vi "PH_BL-Master.get class of status subscriber.vi"(0 "GUI Ref":refnum<vi>, 1 "Ref Switch Instances":refnum<vi>, 2 "Ref BB Instances":refnum<vi>, 3 "Ref 6P Switch Instances":refnum<vi>, 4 "Ref Switch GUI Instances":refnum<vi>, 5 "Ref Switch and 6P State Instances":refnum<vi>, 7 "Force Sensor Instances":refnum<vi>) -> (17 "Status Subscriber Class":T1)   [LabVIEW 2014, in "PH_BL-Master.lvlib"]
uses:
  PH_BL-Master.lvlib
  PH_BL-Master.Status Subscriber Class.ctl
  PH_Basics/PH_Common/PH_Common.lvlib
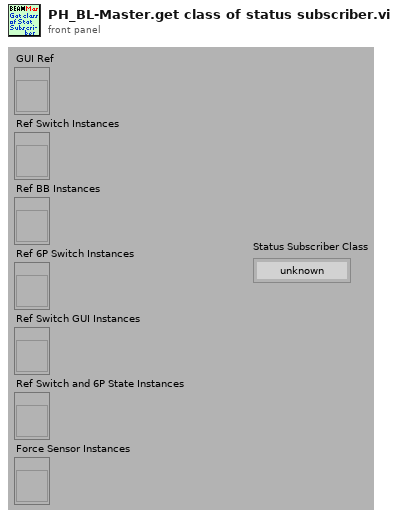
[diagram p1: front panel]
types:
  T1 = typedef "PH_BL-Master.lvlib/PH_BL-Master.Status Subscriber Class.ctl" = enum16{"unknown", "Switch", "BB", "6P Switch", "Switch GUI", "Switch and 6P State", "Force Sensor"}
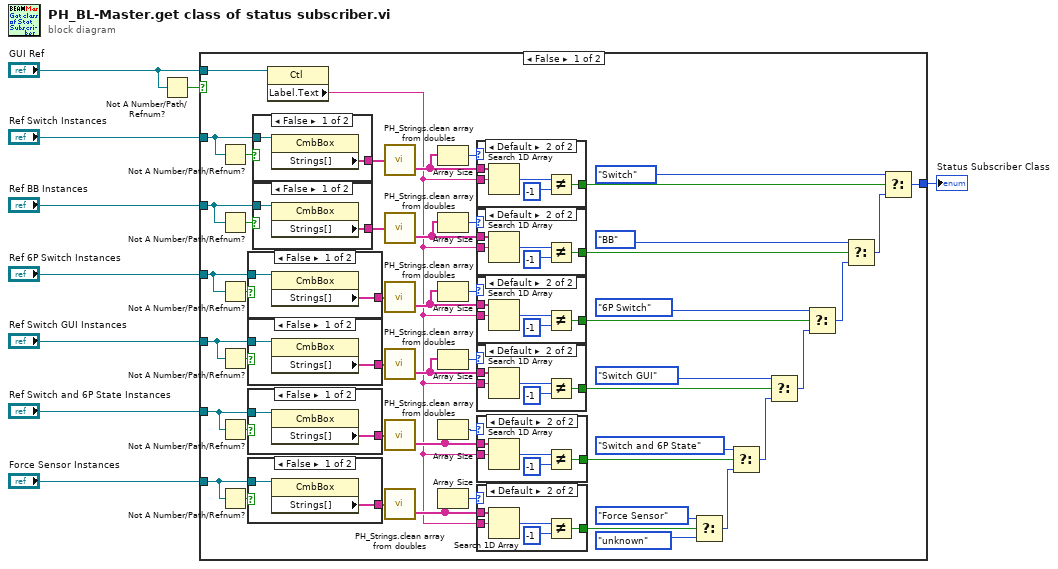
[diagram p0: block diagram]
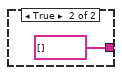
[diagram p2: hidden frame]
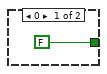
[diagram p3: hidden frame]
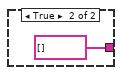
[diagram p4: hidden frame]
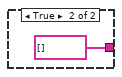
[diagram p5: hidden frame]
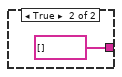
[diagram p6: hidden frame]
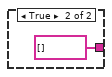
[diagram p7: hidden frame]
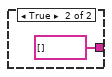
[diagram p8: hidden frame]
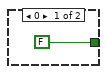
[diagram p9: hidden frame]
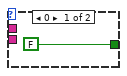
[diagram p10: hidden frame]
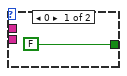
[diagram p11: hidden frame]
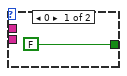
[diagram p12: hidden frame]
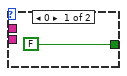
[diagram p13: hidden frame]
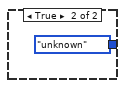
[diagram p14: hidden frame]
diagram:
  n1 = Not A Number/Path/Refnum?(number/path/refnum="GUI Ref") -> (NaN/Path/Refnum?=w2:bool)
  n2 = case shown="False" w2 {
    tunnel: "GUI Ref" -> [w59 _]
    tunnel: [w56 PH_BL-Master.Status_Subscriber_Class."unknown" ("Status Subscriber Class")] -> w9
    tunnel: "Ref Switch Instances" -> [w32 _]
    tunnel: "Ref BB Instances" -> [w23 _]
    tunnel: "Ref 6P Switch Instances" -> [w22 _]
    tunnel: "Ref Switch GUI Instances" -> [w21 _]
    tunnel: "Ref Switch and 6P State Instances" -> [w20 _]
    tunnel: "Force Sensor Instances" -> [w16 _]
    frame False {
      n3 = Not A Number/Path/Refnum?(number/path/refnum=w32) -> (NaN/Path/Refnum?=w33:bool)
      n4 = Not A Number/Path/Refnum?(number/path/refnum=w23) -> (NaN/Path/Refnum?=w31:bool)
      n5 = Not A Number/Path/Refnum?(number/path/refnum=w22) -> (NaN/Path/Refnum?=w30:bool)
      n6 = Not A Number/Path/Refnum?(number/path/refnum=w21) -> (NaN/Path/Refnum?=w29:bool)
      n7 = Not A Number/Path/Refnum?(number/path/refnum=w20) -> (NaN/Path/Refnum?=w28:bool)
      n8 = Not A Number/Path/Refnum?(number/path/refnum=w16) -> (NaN/Path/Refnum?=w18:bool)
      n9 = case shown="False" w30 {
        tunnel: [w77 string[] [] ("Strings[]")] -> w26
        tunnel: w22 -> [w76 _]
        frame False {
          n10 = property class="CmbBox"(reference=w76) -> ("Strings[]"=w77:string[])  [unwired: 1 in, 2 out]
        }
        frame True {
        }
      }
      n11 = case shown="False" w29 {
        tunnel: [w74 string[] [] ("Strings[]")] -> w25
        tunnel: w21 -> [w73 _]
        frame False {
          n12 = property class="CmbBox"(reference=w73) -> ("Strings[]"=w74:string[])  [unwired: 1 in, 2 out]
        }
        frame True {
        }
      }
      n13 = case shown="False" w28 {
        tunnel: [w71 string[] [] ("Strings[]")] -> w24
        tunnel: w20 -> [w70 _]
        frame False {
          n14 = property class="CmbBox"(reference=w70) -> ("Strings[]"=w71:string[])  [unwired: 1 in, 2 out]
        }
        frame True {
        }
      }
      n15 = case shown="False" w18 {
        tunnel: [w62 string[] [] ("Strings[]")] -> w17
        tunnel: w16 -> [w61 _]
        frame False {
          n16 = property class="CmbBox"(reference=w61) -> ("Strings[]"=w62:string[])  [unwired: 1 in, 2 out]
        }
        frame True {
        }
      }
      n17 = case shown="False" w33 {
        tunnel: [w83 string[] [] ("Strings[]")] -> w60
        tunnel: w32 -> [w82 _]
        frame False {
          n18 = property class="CmbBox"(reference=w82) -> ("Strings[]"=w83:string[])  [unwired: 1 in, 2 out]
        }
        frame True {
        }
      }
      n19 = case shown="False" w31 {
        tunnel: [w80 string[] [] ("Strings[]")] -> w27
        tunnel: w23 -> [w79 _]
        frame False {
          n20 = property class="CmbBox"(reference=w79) -> ("Strings[]"=w80:string[])  [unwired: 1 in, 2 out]
        }
        frame True {
        }
      }
      n21 = property class="Ctl"(reference=w59) -> ("Label.Text"=w15:string)  [unwired: 1 in, 2 out]
      n22 = call "PH_Strings.clean array from doubles.vi"("Array Input"=w60) -> ("Cleaned Array Output"=w55:string[])  [unwired: 1 out]
      n23 = call "PH_Strings.clean array from doubles.vi"("Array Input"=w27) -> ("Cleaned Array Output"=w49:string[])  [unwired: 1 out]
      n24 = call "PH_Strings.clean array from doubles.vi"("Array Input"=w26) -> ("Cleaned Array Output"=w48:string[])  [unwired: 1 out]
      n25 = call "PH_Strings.clean array from doubles.vi"("Array Input"=w25) -> ("Cleaned Array Output"=w47:string[])  [unwired: 1 out]
      n26 = call "PH_Strings.clean array from doubles.vi"("Array Input"=w24) -> ("Cleaned Array Output"=w46:string[])  [unwired: 1 out]
      n27 = call "PH_Strings.clean array from doubles.vi"("Array Input"=w17) -> ("Cleaned Array Output"=w19:string[])  [unwired: 1 out]
      n28 = Array Size(array=w55) -> (size(s)=w54:i32)
      n29 = Array Size(array=w49) -> (size(s)=w53:i32)
      n30 = Array Size(array=w48) -> (size(s)=w52:i32)
      n31 = Array Size(array=w47) -> (size(s)=w51:i32)
      n32 = Array Size(array=w46) -> (size(s)=w50:i32)
      n33 = Array Size(array=w19) -> (size(s)=w14:i32)
      n34 = case shown="Default" w54 {
        tunnel: w15 -> [_ w114]
        tunnel: [FALSE w111] -> w58
        tunnel: w55 -> [_ w110]
        frame 0 {
        }
        frame Default {
          n35 = Search 1D Array(1D array=w110, element=w114) -> (index of element=w113:i32)  [unwired: 1 in]
          n36 = Not Equal?(x=w113, y=-1) -> (x != y?=w111:bool)
        }
      }
      n37 = case shown="Default" w53 {
        tunnel: w15 -> [_ w108]
        tunnel: [FALSE w105] -> w45
        tunnel: w49 -> [_ w104]
        frame 0 {
        }
        frame Default {
          n38 = Search 1D Array(1D array=w104, element=w108) -> (index of element=w107:i32)  [unwired: 1 in]
          n39 = Not Equal?(x=w107, y=-1) -> (x != y?=w105:bool)
        }
      }
      n40 = case shown="Default" w52 {
        tunnel: w15 -> [_ w102]
        tunnel: [FALSE w99] -> w44
        tunnel: w48 -> [_ w98]
        frame 0 {
        }
        frame Default {
          n41 = Search 1D Array(1D array=w98, element=w102) -> (index of element=w101:i32)  [unwired: 1 in]
          n42 = Not Equal?(x=w101, y=-1) -> (x != y?=w99:bool)
        }
      }
      n43 = case shown="Default" w51 {
        tunnel: w15 -> [_ w96]
        tunnel: [FALSE w93] -> w43
        tunnel: w47 -> [_ w92]
        frame 0 {
        }
        frame Default {
          n44 = Search 1D Array(1D array=w92, element=w96) -> (index of element=w95:i32)  [unwired: 1 in]
          n45 = Not Equal?(x=w95, y=-1) -> (x != y?=w93:bool)
        }
      }
      n46 = case shown="Default" w50 {
        tunnel: w15 -> [_ w90]
        tunnel: [FALSE w87] -> w42
        tunnel: w46 -> [_ w86]
        frame 0 {
        }
        frame Default {
          n47 = Search 1D Array(1D array=w86, element=w90) -> (index of element=w89:i32)  [unwired: 1 in]
          n48 = Not Equal?(x=w89, y=-1) -> (x != y?=w87:bool)
        }
      }
      n49 = case shown="Default" w14 {
        tunnel: w15 -> [_ w69]
        tunnel: [FALSE w66] -> w13
        tunnel: w19 -> [_ w65]
        frame 0 {
        }
        frame Default {
          n50 = Search 1D Array(1D array=w65, element=w69) -> (index of element=w68:i32)  [unwired: 1 in]
          n51 = Not Equal?(x=w68, y=-1) -> (x != y?=w66:bool)
        }
      }
      n52 = Select(t=PH_BL-Master.Status_Subscriber_Class."Force Sensor", s=w13, f=PH_BL-Master.Status_Subscriber_Class."unknown" ("Status Subscriber Class")) -> (s? t:f=w10:T1)
      n53 = Select(t=PH_BL-Master.Status_Subscriber_Class."Switch and 6P State", s=w42, f=w10) -> (s? t:f=w41:T1)
      n54 = Select(t=PH_BL-Master.Status_Subscriber_Class."Switch GUI", s=w43, f=w41) -> (s? t:f=w40:T1)
      n55 = Select(t=PH_BL-Master.Status_Subscriber_Class."6P Switch", s=w44, f=w40) -> (s? t:f=w39:T1)
      n56 = Select(t=PH_BL-Master.Status_Subscriber_Class."BB", s=w45, f=w39) -> (s? t:f=w38:T1)
      n57 = Select(t=PH_BL-Master.Status_Subscriber_Class."Switch" ("Status Subscriber Class"), s=w58, f=w38) -> (s? t:f=w56:T1)
    }
    frame True {
    }
  }
  "Status Subscriber Class" <- w9
